vi "BallRollDistance.vi"(4 "k_switch":dbl=0.714286, 5 "acc_roll":dbl=-2.4, 6 "vcur":dbl, 7 "acc_slide":dbl=-2.5, 8 "error in (no error)":errorcluster, 9 "vf":dbl, 10 "vi":dbl, 11 "object in":refnum<class "Utilities.lvclass">) -> (0 "error out":errorcluster, 2 "dist":dbl, 3 "object out":refnum<class "Utilities.lvclass">)   [LabVIEW 2024, in "Utilities.lvclass"]
uses:
  Utilities.lvclass
panel:
  out "dist 2":dbl
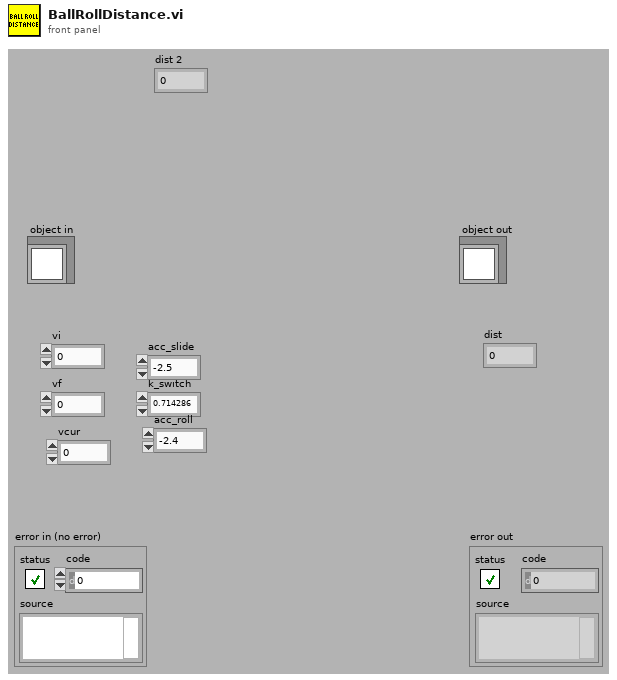
[diagram p1: front panel]
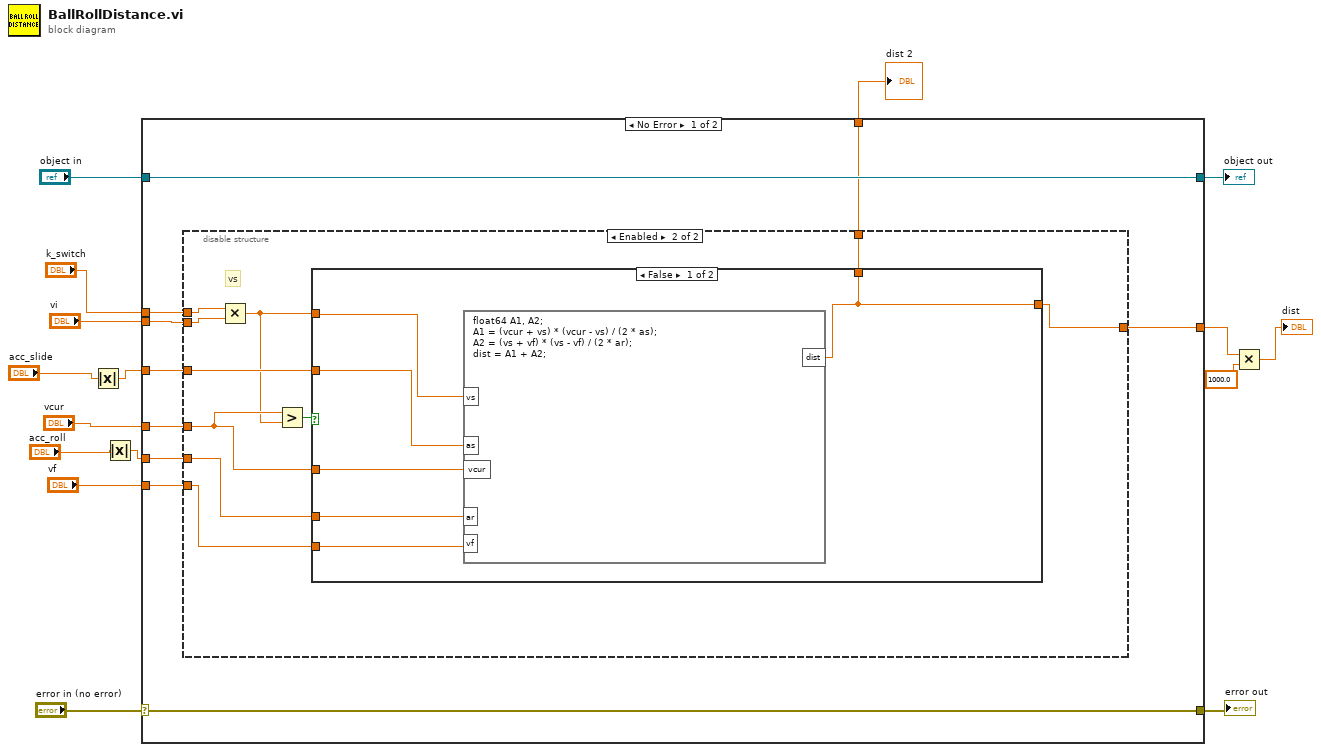
[diagram p0: block diagram]
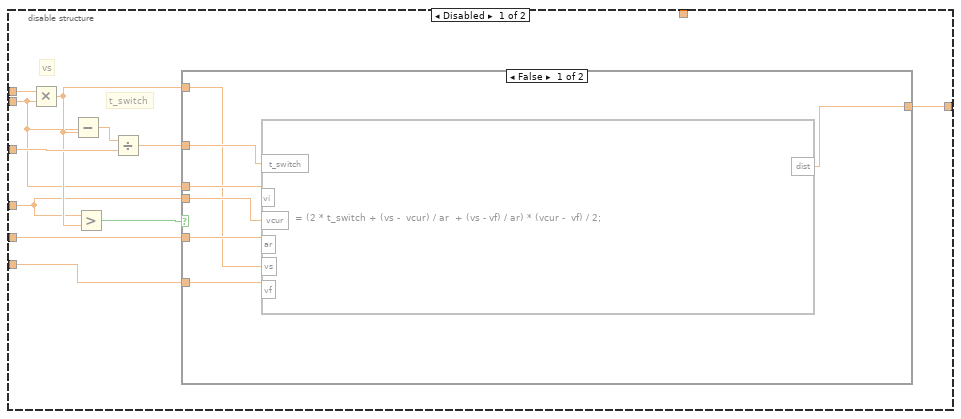
[diagram p2: hidden frame]
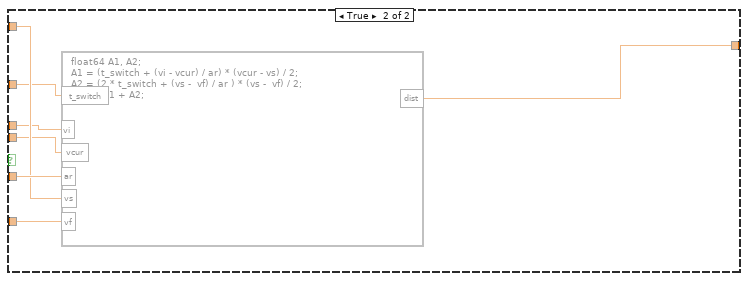
[diagram p3: hidden frame]
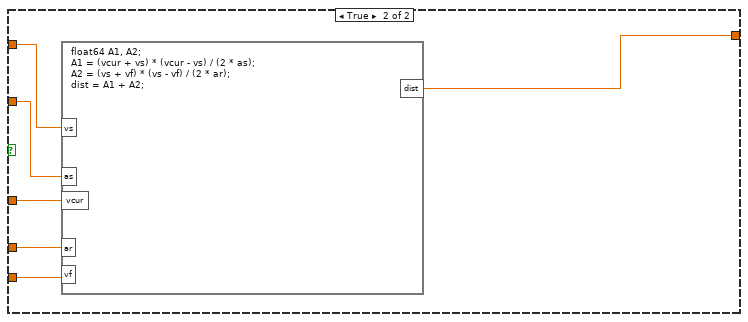
[diagram p4: hidden frame]
diagram:
  n1 = Absolute Value(x="acc_slide") -> (abs(x)=w7:dbl)
  n2 = Absolute Value(x="acc_roll") -> (abs(x)=w5:dbl)
  n3 = case shown="No Error" "error in (no error)" {
    selector: "error in (no error)" -> [w25 w75]
    tunnel: [w25 w75] -> w15
    tunnel: [w26 w74] -> w13
    tunnel: "object in" -> [w26 w74]
    tunnel: "vi" -> [w18 _]
    tunnel: "k_switch" -> [w24 _]
    tunnel: "vcur" -> [w19 _]
    tunnel: w7 -> [w23 _]
    tunnel: [w22 _] -> w4
    tunnel: "vf" -> [w21 _]
    tunnel: w5 -> [w20 _]
    tunnel: [w17 _] -> w1
    frame No Error {
      n4 = disable-structure shown="Enabled" {
        disable-tunnel: w24 -> [w37 w60]
        disable-tunnel: w23 -> [w34 w56]
        disable-tunnel: [w33 w61] -> w22
        disable-tunnel: w21 -> [w32 w59]
        disable-tunnel: w20 -> [w31 w58]
        disable-tunnel: w19 -> [w29 w54]
        disable-tunnel: w18 -> [w28 w57]
        disable-tunnel: [_ w52] -> w17
        frame Disabled {
          # "t_switch"
          # "vs"
          n5 = Multiply(x=w37, y=w28) -> (x*y=w30:dbl)
          n6 = Subtract(x=w28, y=w30) -> (x-y=w35:dbl)
          n7 = Greater?(x=w29, y=w30) -> (0:w36:bool)
          n8 = Divide(x=w35, y=w34) -> (x/y=w27:dbl)
          n9 = case shown="False" w36 {
            tunnel: [w44 w51] -> w33
            tunnel: w32 -> [w38 w50]
            tunnel: w31 -> [w40 w49]
            tunnel: w30 -> [w39 w48]
            tunnel: w29 -> [w41 w47]
            tunnel: w28 -> [w42 w46]
            tunnel: w27 -> [w43 w45]
            frame False {
              n10 = formula code="dist  = (2 * t_switch + (vs -  vcur) / ar  + (vs - vf) / ar) * (vcur -  vf) / 2;"("t_switch"=w43, "vi"=w42, "vcur"=w41, "ar"=w40, "vs"=w39, "vf"=w38) -> ("dist"=w44:dbl)
            }
            frame True {
              n11 = formula code="float64 A1, A2;\nA1 = (t_switch + (vi - vcur) / ar) * (vcur - vs) / 2;\nA2 = (2 * t_switch + (vs -  vf) / ar ) * (vs -  vf) / 2;\ndist = A1 + A2;"("t_switch"=w45, "vi"=w46, "vcur"=w47, "ar"=w49, "vs"=w48, "vf"=w50) -> ("dist"=w51:dbl)
            }
          }
        }
        frame Enabled {
          # "vs"
          n12 = Multiply(x=w60, y=w57) -> (x*y=w53:dbl)
          n13 = Greater?(x=w54, y=w53) -> (0:w55:bool)
          n14 = case shown="False" w55 {
            tunnel: [w62 w73] -> w61
            tunnel: w53 -> [w67 w72]
            tunnel: w59 -> [w63 w71]
            tunnel: w58 -> [w64 w70]
            tunnel: w54 -> [w65 w69]
            tunnel: w56 -> [w66 w68]
            tunnel: [w62 _] -> w52
            frame False {
              n15 = formula code="float64 A1, A2;\nA1 = (vcur + vs) * (vcur - vs) / (2 * as);\nA2 = (vs + vf) * (vs - vf) / (2 * ar);\ndist = A1 + A2;"("as"=w66, "vcur"=w65, "ar"=w64, "vs"=w67, "vf"=w63) -> ("dist"=w62:dbl)
            }
            frame True {
              n16 = formula code="float64 A1, A2;\nA1 = (vcur + vs) * (vcur - vs) / (2 * as);\nA2 = (vs + vf) * (vs - vf) / (2 * ar);\ndist = A1 + A2;"("as"=w68, "vcur"=w69, "ar"=w70, "vs"=w72, "vf"=w71) -> ("dist"=w73:dbl)
            }
          }
        }
      }
    }
    frame Error {
    }
  }
  "error out" <- w15
  "object out" <- w13
  "dist 2" <- w1
  n17 = Multiply(x=w4, y=1000.0) -> (x*y=→"dist":dbl)
